vi "_CSM Module Switcher.vi"(7 "Module Name":string="CSM Debug Console") -> ()   [LabVIEW 2017]
uses:
  user.lib/_NEVSTOP/Communicable State Machine(CSM)/_Support/Typedef/_CSM_GlobalLog_MSG.ctl
  user.lib/_NEVSTOP/Communicable State Machine(CSM)/_Support/Typedef/_CSM_Response Source Message.ctl
  user.lib/_NEVSTOP/Communicable State Machine(CSM)/_Support/Typedef/_CSM_GlobalLog_MSG_TYPE.ctl
  user.lib/_NEVSTOP/Communicable State Machine(CSM)/_Support/Common/Format Timestamp.vi
  user.lib/_NEVSTOP/Communicable State Machine(CSM)/AdvanceAPI/CSM - Convert Error to Argument.vi
  user.lib/_NEVSTOP/Communicable State Machine(CSM)/_Support/GlobalEvent/GEvt-Generate with Rule Check.vi
  user.lib/_NEVSTOP/Communicable State Machine(CSM)/AdvanceAPI/CSM - Keywords.vi
  user.lib/_NEVSTOP/Communicable State Machine(CSM)/AdvanceAPI/CSM - Make String Arguments Safe.vi
  user.lib/_NEVSTOP/Communicable State Machine(CSM)/_Support/GlobalEvent/LogFilter/LogFilter - Check.vi
  user.lib/_NEVSTOP/Communicable State Machine(CSM)/_Support/GlobalEvent/Cache-GEvt Refs.vi
  user.lib/_NEVSTOP/Communicable State Machine(CSM)/_Support/GlobalEvent/LogFilter/LogFilter.lvclass
  user.lib/_NEVSTOP/Communicable State Machine(CSM)/Communicable State Machine.lvlib
  user.lib/_NEVSTOP/Communicable State Machine(CSM)/_tool/_jksm/JKISM Message Event.lvlib
  user.lib/_NEVSTOP/Communicable State Machine(CSM)/_csmHelper/API with lvcsm Support/CSM-Helper API with lvcsm Support.lvlib
  user.lib/_NEVSTOP/Communicable State Machine(CSM)/_Shared/CSM Shared.lvlib
panel:
  in  "Toolbar.Exit":bool
  in  "Toolbar.Refresh lvcsm Cache":bool
  in  "Refresh CSMs Button":bool
  in  "CSM":string(combo)
  in  "Toolbar.Open FP":bool
  in  "Toolbar.Open BD":bool
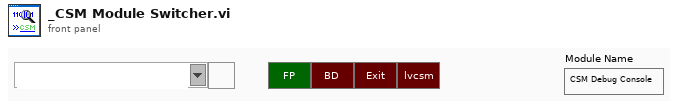
[diagram p1: front panel]
types:
  T1 = typedef "Communicable State Machine.lvlib/_CSM_GlobalLog_MSG.ctl" = cluster{"Name (\"\" to Use UUID)":string, "Current State":string, "Arguments":string, "Source Message":T2, "Source Module":string, "Complete(T)/Start(F)":bool, "LogType":T3, "Time Stamp":timestamp}
  T2 = typedef "Communicable State Machine.lvlib/_CSM_Response Source Message.ctl" = cluster{"‘State":string, "’Arguments":string, "’Error":errorcluster}
  T3 = typedef "Communicable State Machine.lvlib/_CSM_GlobalLog_MSG_TYPE.ctl" = enum16{"User Log", "State Change", "Status", "Interrupt", "Register", "Unregister", "Error Log", "Module Created", "Module Destroyed", "Async Message", "No-Rep Async Message", "Sync Message"}
  T4 = enum32{"Invalid", "Standard", "Closed", "Hidden", "Minimized", "Maximized"}
  T5 = enum32{"invalid app kind", "Development System", "Run Time System", "Student Edition", "Embedded LabVIEW", "Evaluation", "Custom"}
  T6 = cluster{"Shift":bool, "Ctrl":bool, "Alt":bool, "Cmd":bool, "Opt":bool}
  T7 = cluster{"Core":cluster{"Current VI Reference":refnum<vi>, "Close Panel on Exit?":bool}, "lvlps File":path, "Toobar.advance":refnum<vi>[]}
  T8 = cluster{"Current VI Reference":refnum<vi>, "Close Panel on Exit?":bool}
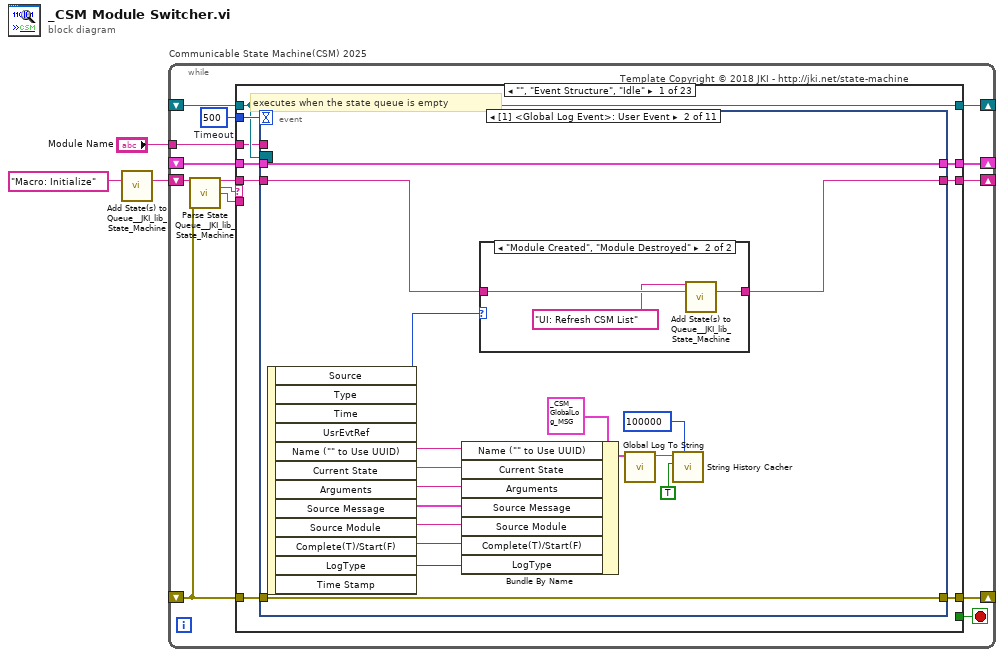
[diagram p0: block diagram]
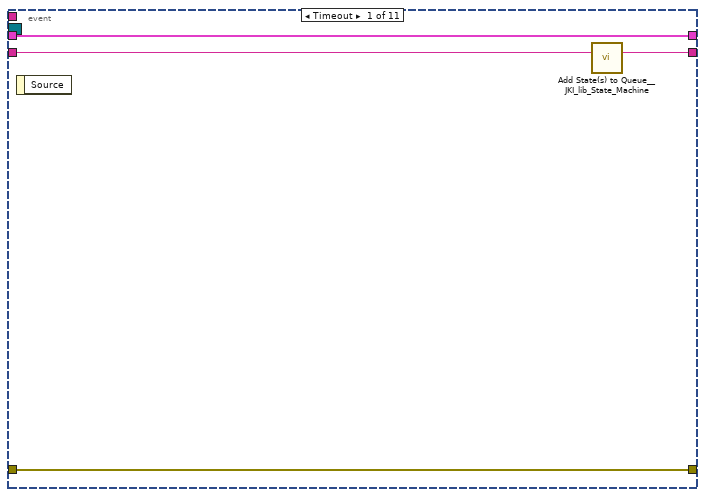
[diagram p2: hidden frame]
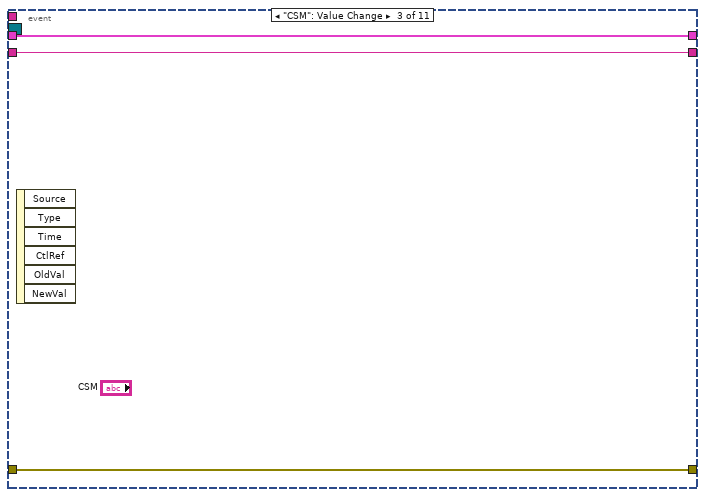
[diagram p4: hidden frame]
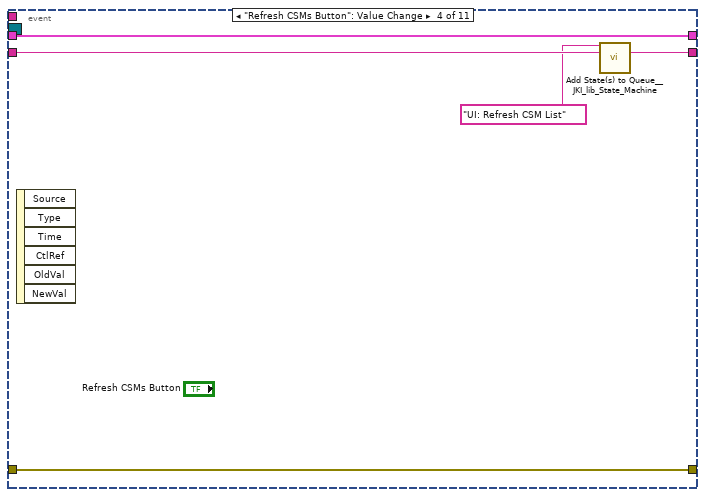
[diagram p5: hidden frame]
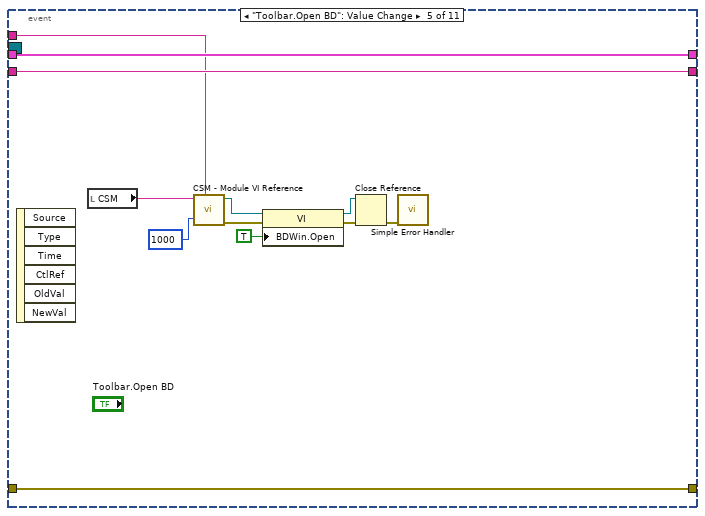
[diagram p6: hidden frame]
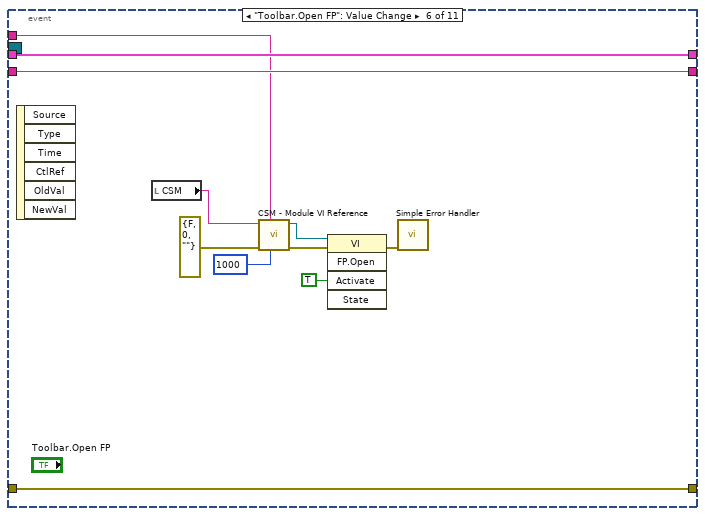
[diagram p7: hidden frame]
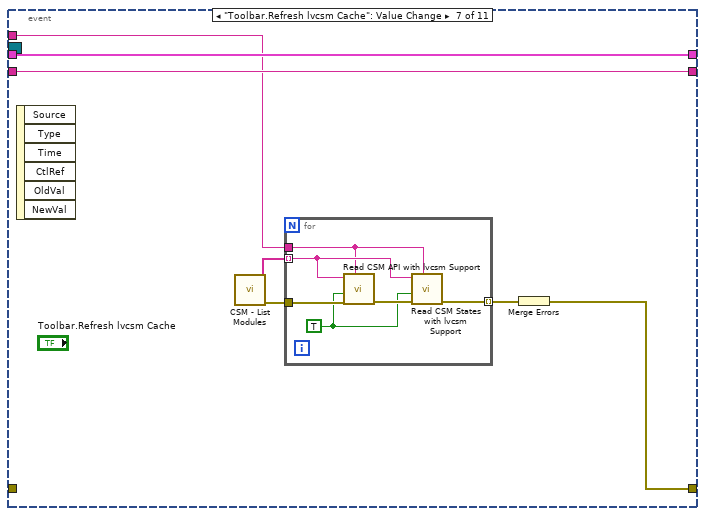
[diagram p8: hidden frame]
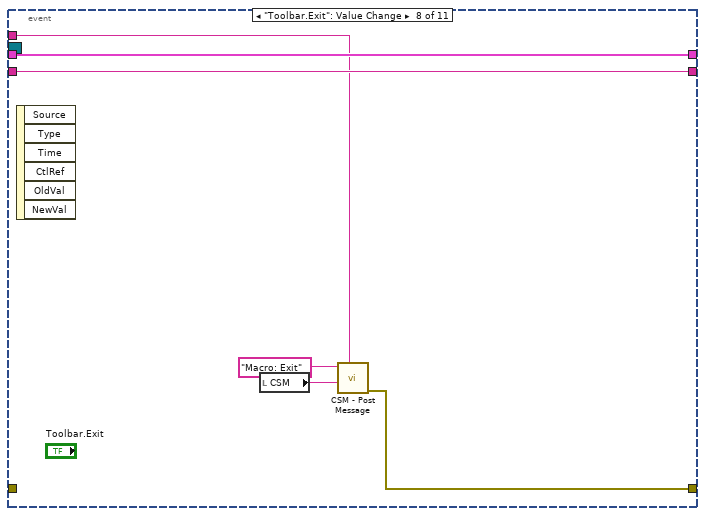
[diagram p9: hidden frame]
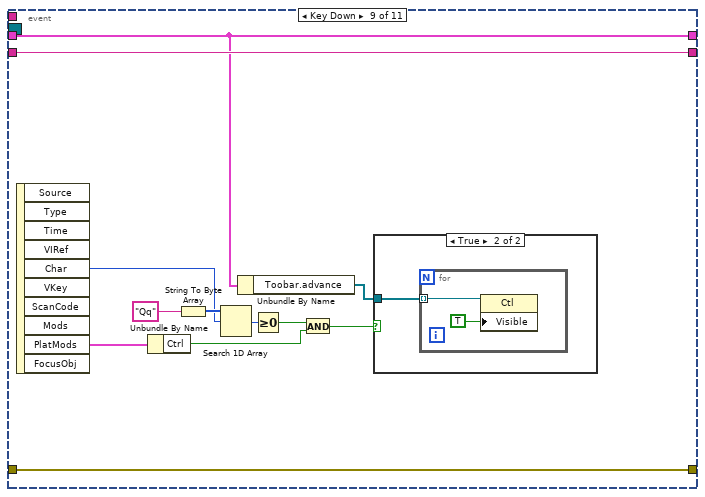
[diagram p10: hidden frame]
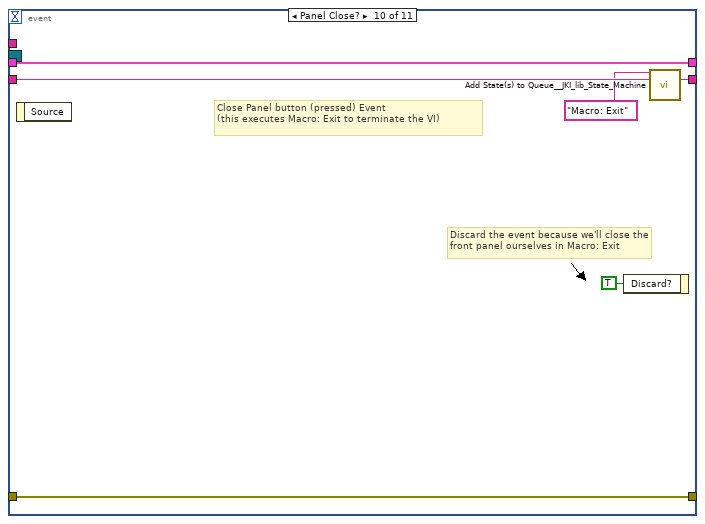
[diagram p12: hidden frame]
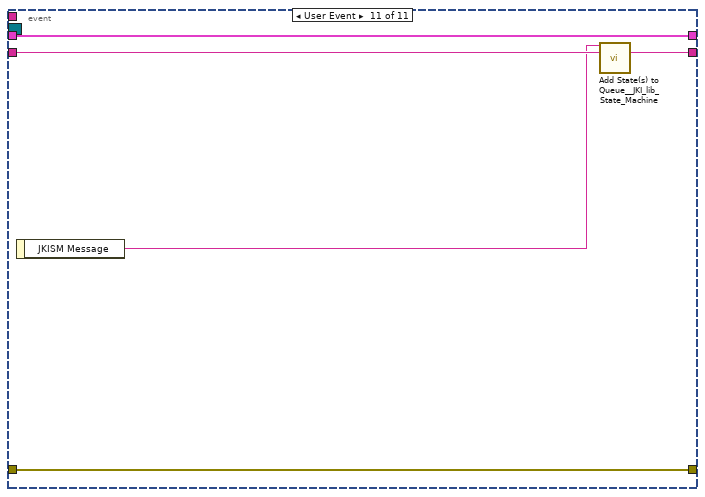
[diagram p13: hidden frame]
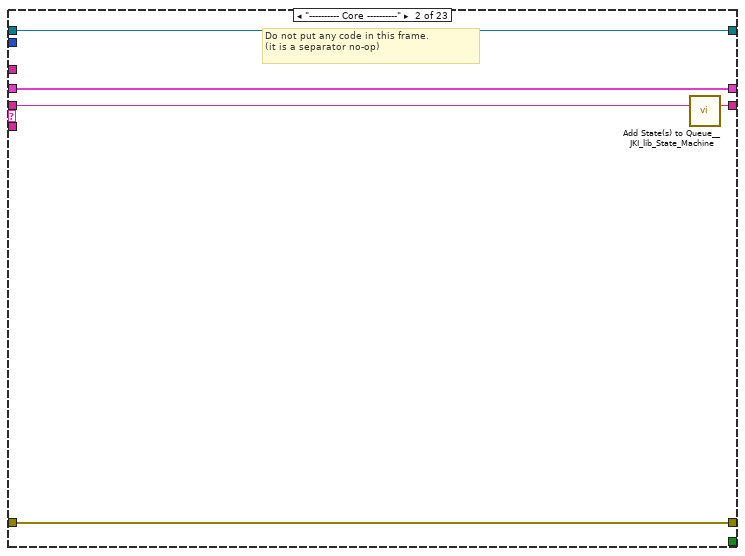
[diagram p14: hidden frame]
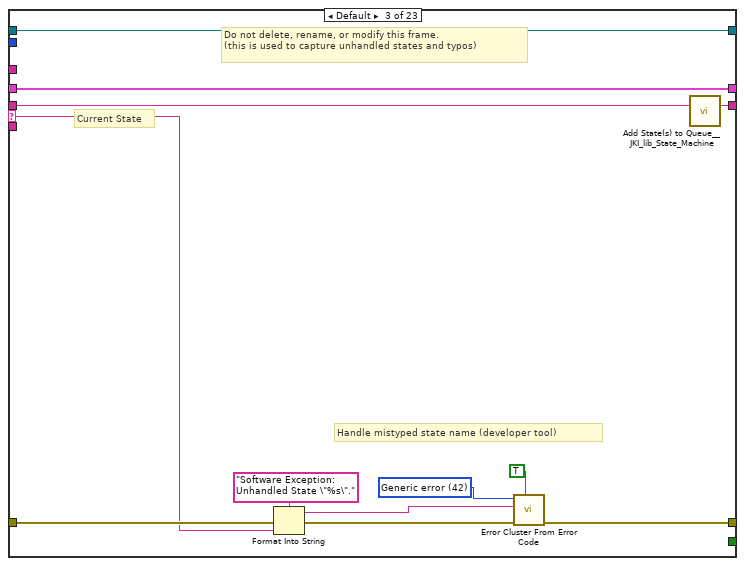
[diagram p15: hidden frame]
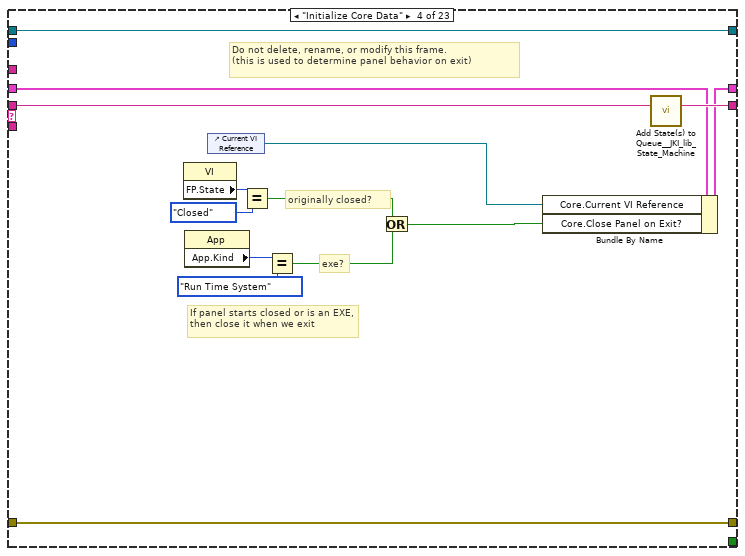
[diagram p16: hidden frame]
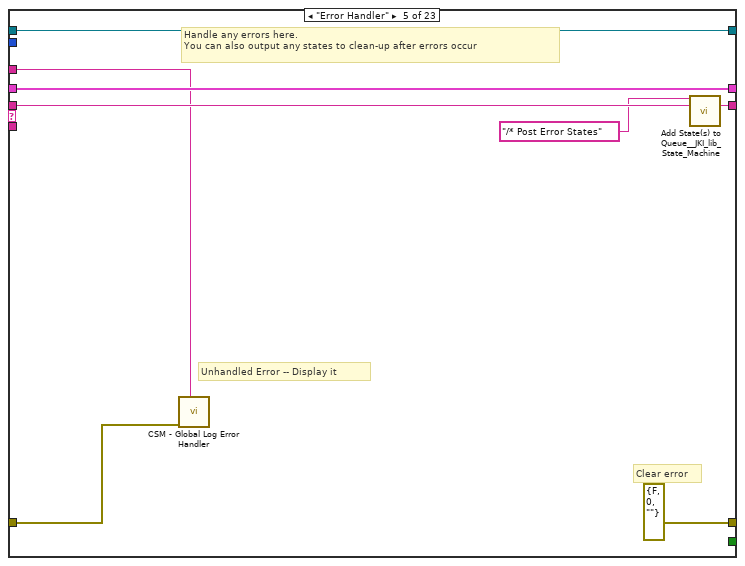
[diagram p17: hidden frame]
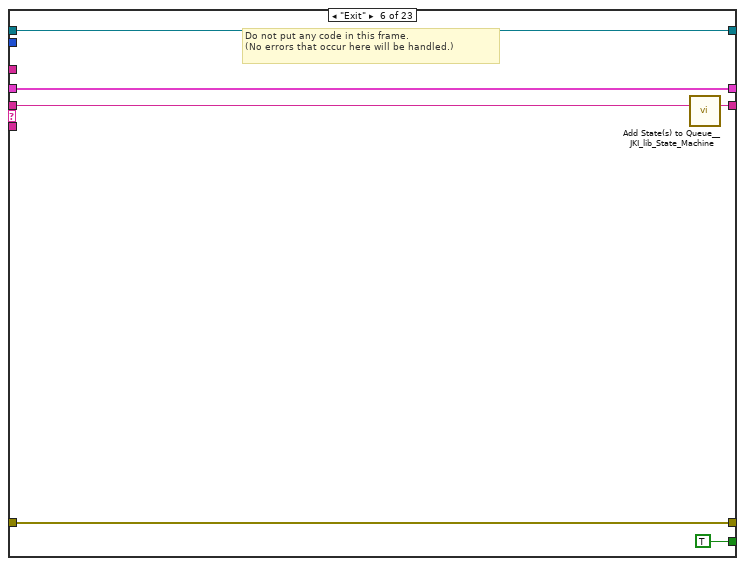
[diagram p18: hidden frame]
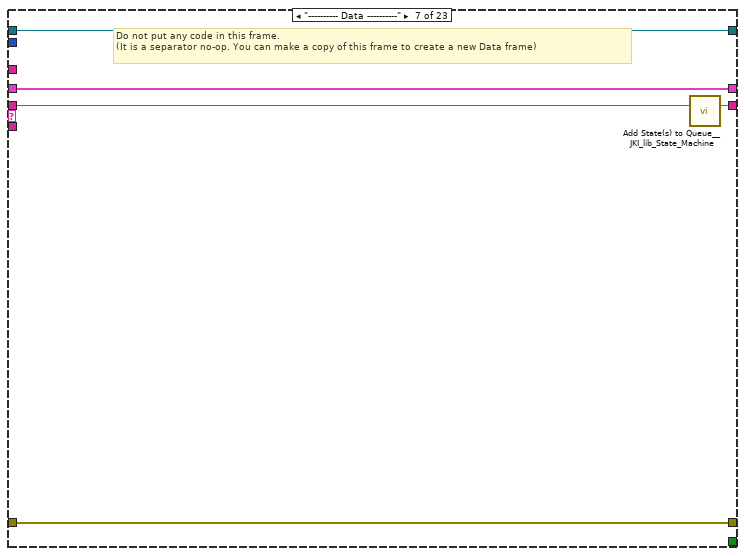
[diagram p19: hidden frame]
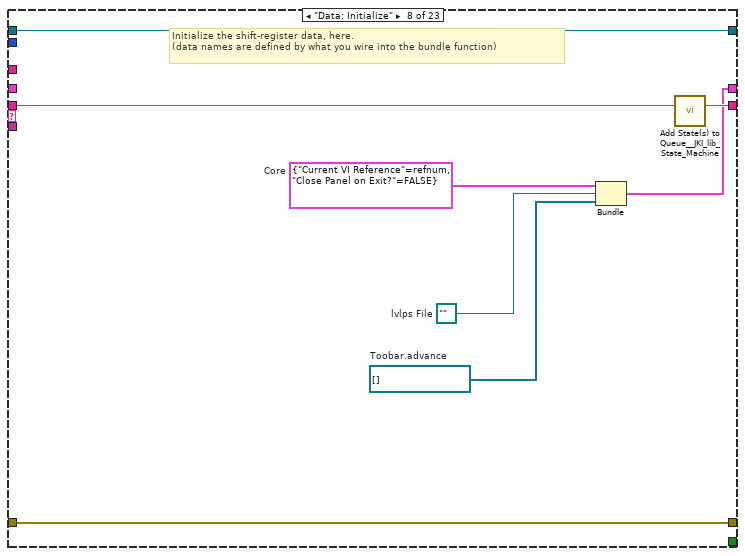
[diagram p20: hidden frame]
diagram:
  n1 = call <vilib>:"Add State(s) to Queue__JKI_lib_State_Machine.vi"("State(s) in (\"\")"="Macro: Initialize") -> ("States Out"=w2:string)  [unwired: 14 in]
  n2 = while "Communicable State Machine(CSM) 2025" {
    shift-right: [w10] -> _
    shift-left: _ -> [w9]
    shift-right: [w13] -> _
    shift-left: _ -> [w7]
    shift-right: [w12] -> _
    shift-left: w2 -> [w14]
    shift-right: [w6] -> _
    shift-left: _ -> [w5]
    tunnel: "Module Name" -> [w4]
    stop <- w11 stop-if-true
    w8 = 500  # Timeout
    # "Template Copyright © 2018 JKI - http://jki.net/state-machine"
    n3 = call <vilib>:"Parse State Queue__JKI_lib_State_Machine.vi"("State Queue"=w14, "Error In (no error)"=w7) -> ("Remaining States"=w16:string, "Current State"=w17:string, "Arguments"=w15:string)  [unwired: 11 in]
    n4 = case shown="\"\", \"Event Structure\", \"Idle\"" w17 {
      selector: w17 -> [_ _ w133 _ _ _ _ _ _ _ _ _ _ _ _ _ _ _ _ _ _ _ _]
      tunnel: w16 -> [w26 w131 w137 w157 w165 w171 w176 w184 w191 w199 w204 w212 w217 w222 w228 w238 w250 w327 w342 w346 w352 w358 w369]
      tunnel: w15 -> [_ _ _ _ _ _ _ _ _ _ _ _ _ _ _ w233 w244 w325 _ _ _ _ _]
      tunnel: w9 -> [w24 w128 w135 w150 w162 w169 w173 _ w190 w194 w201 w210 w213 w219 w224 w236 w246 w322 w341 w344 w349 w355 w366]
      tunnel: [w23 w129 w139 w154 errorcluster {"status"=FALSE, "code"=0, "source"=""} ("error out") w168 w174 w181 w192 w195 w202 w208 w214 w220 w226 w234 w247 w328 w343 w347 w350 w356 w367] -> w13
      tunnel: w7 -> [w22 w129 w138 w154 w161 w168 w174 w181 w192 w196 w202 _ _ w220 w226 w235 w248 w328 w343 w347 w350 w356 w367]
      tunnel: [w25 w130 w136 w156 w164 w170 w175 w183 w191 w198 w203 w211 w216 w221 w227 w237 w249 w327 w342 w346 w351 w357 w368] -> w12
      tunnel: [_ _ _ _ _ TRUE _ _ _ _ _ _ _ _ _ _ _ _ _ _ _ _ _] -> w11
      tunnel: [w21 w128 w135 w155 w162 w169 w173 w182 w186 w194 w201 w210 w213 w219 w224 w236 w246 w322 w341 w344 w349 w355 w366] -> w10
      tunnel: w8 -> [w20 _ _ _ _ _ _ _ _ _ _ _ _ _ _ _ _ _ _ _ _ _ _]
      tunnel: [w19 w127 w132 w144 w159 w166 w172 w179 w189 w193 w200 w209 w215 w218 w225 w232 w243 w326 w340 w345 w348 w353 w359] -> w6
      tunnel: w5 -> [w19 w127 w132 w144 w159 w166 w172 w179 w189 w193 w200 _ w215 w218 w225 w232 w243 w326 w340 w345 w348 w353 w359]
      tunnel: w4 -> [w18 _ _ _ w158 _ _ _ _ _ _ w205 _ _ _ _ _ _ _ _ _ _ _]
      frame "", "Event Structure", "Idle" {
        # "executes when the state queue is empty"
        n5 = event shown="[1] <Global Log Event>: User Event" {
          selector: w19 -> [_ _ _ _ _ _ _ _ _ _ _]
          dyn-events: _ -> [_ _ _ _ _ _ _ _ _ _ _]
          timeout: w20 -> [_ _ _ _ _ _ _ _ _ _ _]
          tunnel: w26 -> [w30 w32 w53 w56 w70 w81 w88 w100 w112 w121 w123]
          tunnel: [w29 w33 w53 w55 w70 w81 w88 w100 w112 w120 w124] -> w25
          tunnel: w24 -> [w27 w45 w51 w57 w69 w80 w87 w99 w101 w118 w125]
          tunnel: [w28 w46 w52 w58 w66 w78 w82 w97 w111 w119 w126] -> w23
          tunnel: w22 -> [w28 w46 w52 w58 w66 w78 _ _ w111 w119 w126]
          tunnel: [w27 w45 w51 w57 w69 w80 w87 w99 w101 w118 w125] -> w21
          tunnel: w18 -> [_ _ _ _ w65 w76 w83 w95 _ _ _]
          event Timeout {
            n6 = event-data() -> ()  [unwired: 1 in, 1 out]
            n7 = call <vilib>:"Add State(s) to Queue__JKI_lib_State_Machine.vi"("State(s) in (\"\")"=w30) -> ("States Out"=w29:string)  [unwired: 14 in]
          }
          event User Event {
            n8 = event-data() -> ("Name (\"\" to Use UUID)"=w39:string, "Current State"=w38:string, "Arguments"=w37:string, "Source Message"=w36:T2, "Source Module"=w35:string, "Complete(T)/Start(F)"=w34:bool, "LogType"=w31:T3)  [unwired: 1 in, 5 out]
            n9 = Bundle By Name(cluster=T1 {"Name (\"\" to Use UUID)"="", "Current State"="", "Arguments"="", "Source Message"={"‘State"="", "’Arguments"="", "’Error"={"status"=FALSE, "code"=0, "source"=""}}, "Source Module"="", "Complete(T)/Start(F)"=FALSE, "LogType"=enum."User Log", "Time Stamp"=timestamp(0 s since 1904-01-01)} ("Cross CSM Data"), "Name (\"\" to Use UUID)"=w39, "Current State"=w38, "Arguments"=w37, "Source Message"=w36, "Source Module"=w35, "Complete(T)/Start(F)"=w34, "LogType"=w31) -> (w44:T1)
            n10 = case shown="\"Module Created\", \"Module Destroyed\"" w31 {
              tunnel: w32 -> [w47 w50]
              tunnel: [w47 w49] -> w33
              frame "User Log", Default {
              }
              frame "Module Created", "Module Destroyed" {
                n11 = call <vilib>:"Add State(s) to Queue__JKI_lib_State_Machine.vi"("State(s) in Front (\"\")"="UI: Refresh CSM List" ("State(s) in Front (\"\")"), "State(s) in (\"\")"=w50) -> ("States Out"=w49:string)  [unwired: 13 in]
              }
            }
            n12 = call "Global Log To String.vi"("Log"=w44) -> ("Log String"=w43:string)  [unwired: 9 in]
            n13 = call "String History Cacher.vi"("Length"=100000 ("length"), "Include Timestamp? (T)"=TRUE ("Include Timestamp(F)"), "String"=w43) -> ()  [unwired: 8 in, 1 out]
          }
          event "CSM": Value Change {
            n14 = event-data() -> ()  [unwired: 1 in, 6 out]
          }
          event "Refresh CSMs Button": Value Change {
            n15 = event-data() -> ()  [unwired: 1 in, 6 out]
            n16 = call <vilib>:"Add State(s) to Queue__JKI_lib_State_Machine.vi"("State(s) in Front (\"\")"="UI: Refresh CSM List" ("State(s) in Front (\"\")"), "State(s) in (\"\")"=w56) -> ("States Out"=w55:string)  [unwired: 13 in]
          }
          event "Toolbar.Open BD": Value Change {
            n17 = event-data() -> ()  [unwired: 1 in, 6 out]
            n18 = local read "CSM"() -> (w67:string)
            n19 = call "CSM - Module VI Reference.vi"("Response Timeout (-2 Using Global Settings)"=1000 ("Response Timeout(5000ms)"), "Current Module (\"\" to Generate an ID)"=w65, "CSM Name"=w67) -> ("error out"=w59:errorcluster, "CSM Module VIRef"=w64:refnum<vi>)  [unwired: 7 in]
            n20 = property class="VI"(reference=w64, error in=w59, "BDWin.Open"=TRUE ("Block Diagram Window:Open")) -> (reference out=w62:refnum<vi>, error out=w61:errorcluster)
            n21 = Close Reference(reference=w62, error in (no error)=w61) -> (error out=w68:errorcluster)
            n22 = call <vilib>:"Simple Error Handler.vi"("error in (no error)"=w68) -> ()  [unwired: 4 in, 5 out]
          }
          event "Toolbar.Open FP": Value Change {
            n23 = event-data() -> ()  [unwired: 1 in, 6 out]
            n24 = local read "CSM"() -> (w79:string)
            n25 = call "CSM - Module VI Reference.vi"("Response Timeout (-2 Using Global Settings)"=1000 ("Response Timeout(5000ms)"), "Current Module (\"\" to Generate an ID)"=w76, "error in (no error)"=errorcluster {"status"=FALSE, "code"=0, "source"=""}, "CSM Name"=w79) -> ("error out"=w72:errorcluster, "CSM Module VIRef"=w73:refnum<vi>)  [unwired: 6 in]
            n26 = invoke on="Invoke Node" class="VI" method="FP.Open"(reference=w73, error in=w72, "Activate"=TRUE ("Activate?")) -> (error out=w77:errorcluster)  [unwired: 2 in, 4 out]
            n27 = call <vilib>:"Simple Error Handler.vi"("error in (no error)"=w77) -> ()  [unwired: 4 in, 5 out]
          }
          event "Toolbar.Refresh lvcsm Cache": Value Change {
            n28 = event-data() -> ()  [unwired: 1 in, 6 out]
            n29 = call "CSM - List Modules.vi"() -> ("error out"=w86:errorcluster, "Module Names"=w85:string[])  [unwired: 10 in]
            n30 = for {
              tunnel: w86 -> [w94]
              tunnel: w85 -> [w92] mode=indexing
              tunnel: w83 -> [w91]
              tunnel: [w90] -> w84 mode=indexing
              w89 = TRUE ("Force?(F)")
              n31 = call "Read CSM API with lvcsm Support.vi"("Current Module (\"\" to Generate an ID)"=w91, "error in (no error)"=w94, "Force? (F)"=w89, "CSM Name"=w92) -> ("error out"=w93:errorcluster)  [unwired: 6 in, 1 out]
              n32 = call "Read CSM States with lvcsm Support.vi"("Current Module (\"\" to Generate an ID)"=w91, "error in (no error)"=w93, "Force? (F)"=w89, "CSM Name"=w92) -> ("error out"=w90:errorcluster)  [unwired: 6 in, 1 out]
            }
            n33 = Merge Errors(w84) -> (w82:errorcluster)
          }
          event "Toolbar.Exit": Value Change {
            n34 = event-data() -> ()  [unwired: 1 in, 6 out]
            n35 = local read "CSM"() -> (w98:string)
            n36 = call "CSM - Post Message.vi"("Current Module (\"\" to Generate an ID)"=w95, "Target Module"=w98, "State"="Macro: Exit") -> ("error out"=w97:errorcluster)  [unwired: 8 in]
          }
          event Key Down {
            n37 = event-data() -> ("Char"=w102:i16, "PlatMods"=w103:T6)  [unwired: 1 in, 8 out]
            n38 = Unbundle By Name(w103) -> ("Ctrl"=w106:bool)
            n39 = String To Byte Array(string="Qq") -> (unsigned byte array=w108:u8[])
            n40 = Search 1D Array(1D array=w108, element=w102) -> (index of element=w109:i32)  [unwired: 1 in]
            n41 = Unbundle By Name(w101) -> ("Toobar.advance"=w104:refnum<vi>[])
            n42 = Greater Or Equal To 0?(x=w109) -> (x >= 0?=w110:bool)
            n43 = And(x=w110, y=w106) -> (x .and. y?=w105:bool)
            n44 = case shown="True" w105 {
              tunnel: w104 -> [_ w113]
              frame False {
              }
              frame True {
                n45 = for {
                  tunnel: w113 -> [w115] mode=indexing
                  n46 = property class="Ctl"(reference=w115, "Visible"=TRUE) -> ()  [unwired: 1 in, 2 out]
                }
              }
            }
          }
          event Panel Close? {
            # "Discard the event because we'll close the front panel ourselves in Macro: Exit"
            # "Close Panel button (pressed) Event\n(this executes Macro: Exit to terminate the VI)"
            n47 = event-data() -> ()  [unwired: 1 in, 1 out]
            n48 = event-data("Discard?"=TRUE) -> ()  [unwired: 1 in, 1 out]
            n49 = call <vilib>:"Add State(s) to Queue__JKI_lib_State_Machine.vi"("State(s) in Front (\"\")"="Macro: Exit", "State(s) in (\"\")"=w121) -> ("States Out"=w120:string)  [unwired: 13 in]
          }
          event User Event {
            n50 = event-data() -> ("JKISM Message"=w122:string)  [unwired: 1 in]
            n51 = call <vilib>:"Add State(s) to Queue__JKI_lib_State_Machine.vi"("State(s) in Front (\"\")"=w122, "State(s) in (\"\")"=w123) -> ("States Out"=w124:string)  [unwired: 13 in]
          }
        }
      }
      frame "---------- Core ----------" {
        # "Do not put any code in this frame.\n(it is a separator no-op)"
        n52 = call <vilib>:"Add State(s) to Queue__JKI_lib_State_Machine.vi"("State(s) in (\"\")"=w131) -> ("States Out"=w130:string)  [unwired: 14 in]
      }
      frame Default {
        w142 = 42 items=["No error", "Argument error", "Memory is full", "Out of zone", "End of file", "File already open", "Generic file I/O error", "File not found", "File permission error", "Disk is full", "Duplicate path", "Too many files open", "System feature not enabled", "Resource file not found", "Cannot add resource", "Resource not found", "Image not found", "Image memory error", "Pen does not exist", "Config type invalid", "Config token not found", "Config parse error", "Config memory error", "Bad external code format", "Bad external code offset", "External code not present", "Null window", "Destroy window error", "Null menu", "Print aborted", "Bad print record", "Print driver error", "Windows error during printing", "Memory error during printing", "Print dialog error", "Generic print error", "Invalid device refnum", "Device not found", "Device parameter error", "Device unit error", "Cannot open device", "Device call aborted", "Generic error", "Cancelled by user", "Object ID too low", "Object ID too high", "Object not in heap", "Unknown heap", "Unknown object (invalid DefProc)", "Unknown object (DefProc not in table)", "Message out of range", "Invalid (null) method", "Unknown message", "Manager call not supported", "Bad address", "Network operation in progress", "Network operation timed out", "Connection is busy", "Network attribute not supported", "Network error", "Address in use", "System out of memory", "Connection aborted", "Connection refused", "Not connected", "Already connected", "Connection closed", "Initialization error (interapplication manager)", "Bad occurrence", "Wait on unbound occurrence handler", "Occurrence queue overflow", "Datalog type conflict", "Unused", "Unrecognized type (interapplication manager)", "Memory corrupt", "Failed to make temporary DLL", "Old CIN version", "Drag socket not found", "Failed to load drop-object", "Failed to register OLE object", "Failed to release OLE object", "Format specifier type mismatch", "Unknown format specifier", "Too few format specifiers", "Too many format specifiers", "Scan failed", "Newer CIN version", "Error converting to variant", "Runtime menu error", "Password tampered", "Variant attribute not found", "Incompatible variant data type", "Event data is not available", "Event Store is not present", "Occurrence is not found", "Event Queue is not created", "Event info is not available", "Refnum passed is NULL", "Error retrieving Class GUID", "Error retrieving CoClass GUID", "Error retrieving TypeLib GUID.", "Bad built application magic bytes.", "Specific driver is different from the specific driver associated with the Logical Name.", "There is no session opened to the class driver.", "Max Error", "MAX - Error with config objects", "MAX - Error loading configuration", "MAX - Group not supported"]
        # "Current State"
        # "Do not delete, rename, or modify this frame.\n(this is used to capture unhandled states and typos)"
        # "Handle mistyped state name (developer tool)"
        n53 = Format Into String(format string="Software Exception: Unhandled State \"%s\"." ("message"), error in=w138, w133) -> (resulting string=w141:string, error out=w140:errorcluster)  [unwired: 1 in]
        n54 = call <vilib>:"Error Cluster From Error Code.vi"("show call chain? (False)"=TRUE, "error in (no error)"=w140, "error message (\"\")"=w141, "error code (0)"=w142) -> ("error out"=w139:errorcluster)  [unwired: 5 in]
        n55 = call <vilib>:"Add State(s) to Queue__JKI_lib_State_Machine.vi"("State(s) in (\"\")"=w137) -> ("States Out"=w136:string)  [unwired: 14 in]
      }
      frame "Initialize Core Data" {
        # "Do not delete, rename, or modify this frame.\n(this is used to determine panel behavior on exit)"
        # "originally closed?"
        # "exe?"
        # "If panel starts closed or is an EXE, then close it when we exit"
        n56 = property class="VI"() -> ("FP.State"=w147:T4)  [unwired: 2 in, 2 out]
        n57 = property class="App"() -> ("App.Kind"=w153:T5)  [unwired: 2 in, 2 out]
        n58 = control-ref of="Current VI Reference"() -> (w148:refnum<vi>)
        n59 = Equal?(x=w147, y=T4."Closed" ("Front Panel Window:State")) -> (x = y?=w145:bool)
        n60 = Equal?(x=w153, y=T5."Run Time System" ("Application:Kind")) -> (x = y?=w151:bool)
        n61 = Or(x=w145, y=w151) -> (x .or. y?=w149:bool)
        n62 = Bundle By Name(cluster=w150, "Core.Current VI Reference"=w148, "Core.Close Panel on Exit?"=w149) -> (w155:T7)
        n63 = call <vilib>:"Add State(s) to Queue__JKI_lib_State_Machine.vi"("State(s) in (\"\")"=w157) -> ("States Out"=w156:string)  [unwired: 14 in]
      }
      frame "Error Handler" {
        # "Unhandled Error -- Display it"
        # "Handle any errors here.\nYou can also output any states to clean-up after errors occur"
        # "Clear error"
        n64 = call "CSM - Global Log Error Handler.vi"("Place (\"\" to Use VI's Name)"=w158, "Error In"=w161) -> ()  [unwired: 9 in, 1 out]
        n65 = call <vilib>:"Add State(s) to Queue__JKI_lib_State_Machine.vi"("State(s) in Front (\"\")"="/* Post Error States", "State(s) in (\"\")"=w165) -> ("States Out"=w164:string)  [unwired: 13 in]
      }
      frame "Exit" {
        # "Do not put any code in this frame.\n(No errors that occur here will be handled.)"
        n66 = call <vilib>:"Add State(s) to Queue__JKI_lib_State_Machine.vi"("State(s) in (\"\")"=w171) -> ("States Out"=w170:string)  [unwired: 14 in]
      }
      frame "---------- Data ----------" {
        # "Do not put any code in this frame.\n(It is a separator no-op. You can make a copy of this frame to create a new Data frame)"
        n67 = call <vilib>:"Add State(s) to Queue__JKI_lib_State_Machine.vi"("State(s) in (\"\")"=w176) -> ("States Out"=w175:string)  [unwired: 14 in]
      }
      frame "Data: Initialize" {
        w177 = refnum<vi>[] []  # Toobar.advance
        w178 = path ""  # lvlps File
        w180 = T8 {"Current VI Reference"=refnum, "Close Panel on Exit?"=FALSE}  # Core
        # "Initialize the shift-register data, here.\n(data names are defined by what you wire into the bundle function)"
        n68 = Bundle("Core"=w180, "lvlps File"=w178, "Toobar.advance"=w177) -> (w182:T7)  [unwired: 1 in]
        n69 = call <vilib>:"Add State(s) to Queue__JKI_lib_State_Machine.vi"("State(s) in (\"\")"=w184) -> ("States Out"=w183:string)  [unwired: 14 in]
      }
      frame "Data: Initialize References" {
        n70 = control-ref of="Toolbar.Open FP"() -> (w188:refnum<vi>)
        n71 = control-ref of="Toolbar.Open BD"() -> (w187:refnum<vi>)
        n72 = Build Array(w188, w187) -> (w185:refnum<vi>[])
        n73 = Bundle By Name(cluster=w190, "Toobar.advance"=w185) -> (w186:T7)
      }
      frame "Data: Cleanup" {
        # "Cleanup any data and references, here.\n(this is called automatically, by the Macro: Exit)"
        n74 = Unbundle By Name(w194) -> ("Core.Current VI Reference"=w197:refnum<vi>)
        n75 = Close Reference(reference=w197, error in (no error)=w196) -> (error out=w195:errorcluster)
        n76 = call <vilib>:"Add State(s) to Queue__JKI_lib_State_Machine.vi"("State(s) in (\"\")"=w199) -> ("States Out"=w198:string)  [unwired: 14 in]
      }
      frame "---------- Events ----------" {
        # "Do not put any code in this frame.\n(It is a separator no-op. You can make a copy of this frame to create a new UI frame)"
        n77 = call <vilib>:"Add State(s) to Queue__JKI_lib_State_Machine.vi"("State(s) in (\"\")"=w204) -> ("States Out"=w203:string)  [unwired: 14 in]
      }
      frame "Events: Register" {
        # "Do not put any code in this frame.\n(It is a separator no-op. You can make a copy of this frame to create a new UI frame)"
        n78 = call "CSM - Global Log Event.vi"() -> ("Global Log Event"=w207:refnum<user-event>)  [unwired: 10 in, 1 out]
        n79 = call "Obtain JKISM Message Event.vi"("Module"=w205) -> ("JKISM Message Event"=w206:refnum<user-event>)  [unwired: 9 in, 1 out]
        n80 = register-events(w207, w206) -> (reference out=w209:refnum<event-registration>, error out=w208:errorcluster)  [unwired: 2 in]
        n81 = call <vilib>:"Add State(s) to Queue__JKI_lib_State_Machine.vi"("State(s) in (\"\")"=w212) -> ("States Out"=w211:string)  [unwired: 14 in]
      }
      frame "Events: Unregister" {
        # "Do not put any code in this frame.\n(It is a separator no-op. You can make a copy of this frame to create a new UI frame)"
        n82 = Unregister For Events(event registration refnum=w215) -> (error out=w214:errorcluster)  [unwired: 1 in]
        n83 = call <vilib>:"Add State(s) to Queue__JKI_lib_State_Machine.vi"("State(s) in (\"\")"=w217) -> ("States Out"=w216:string)  [unwired: 14 in]
      }
      frame "---------- UI ----------" {
        # "Do not put any code in this frame.\n(It is a separator no-op. You can make a copy of this frame to create a new UI frame)"
        n84 = call <vilib>:"Add State(s) to Queue__JKI_lib_State_Machine.vi"("State(s) in (\"\")"=w222) -> ("States Out"=w221:string)  [unwired: 14 in]
      }
      frame "UI: Initialize" {
        # "Initialize the User Interface, here.\n(this is called automatically, by the Macro: Init)"
        n85 = Unbundle By Name(w224) -> ("Toobar.advance"=w223:refnum<vi>[])
        n86 = disable-structure shown="Disabled" {
          disable-tunnel: w223 -> [w229 _]
          frame Disabled {
            n87 = for {
              tunnel: w229 -> [w231] mode=indexing
              n88 = property class="Ctl"(reference=w231, "Visible"=FALSE) -> ()  [unwired: 1 in, 2 out]
            }
          }
          frame Enabled {
          }
        }
        n89 = call <vilib>:"Add State(s) to Queue__JKI_lib_State_Machine.vi"("State(s) in (\"\")"=w228) -> ("States Out"=w227:string)  [unwired: 14 in]
      }
      frame "UI: Cursor Set" {
        # "Argument"
        # "Set and Unset Cursor Busy.\n(Usage: \"UI: Cursor Set >> Busy|Idle\")"
        n90 = case shown="\"Idle\", Default" w233 {
          tunnel: w235 -> [w240 w242]
          tunnel: [w239 w241] -> w234
          frame "Idle", Default {
            n91 = call <vilib>:"Unset Busy.vi"("error in (no error)"=w240) -> ("error out"=w239:errorcluster)  [unwired: 10 in]
          }
          frame "Busy" {
            n92 = call <vilib>:"Set Busy.vi"("error in (no error)"=w242) -> ("error out"=w241:errorcluster)  [unwired: 9 in, 1 out]
          }
        }
        n93 = call <vilib>:"Add State(s) to Queue__JKI_lib_State_Machine.vi"("State(s) in (\"\")"=w238) -> ("States Out"=w237:string)  [unwired: 14 in]
      }
      frame "UI: Front Panel State" {
        # "Argument"
        # "Set Front Panel Open or Closed\n(Usage: \"UI: Front Panel State >> Open|Close\")"
        n94 = Unbundle By Name(w246) -> ("Core.Current VI Reference"=w245:refnum<vi>)
        n95 = case shown="\"Minimize\", \"Minimized\"" w244 {
          tunnel: w248 -> [w256 w271 w282 w295 w308]
          tunnel: [w258 w272 w284 w297 w310] -> w247
          tunnel: w245 -> [w257 w269 w283 w296 w309]
          frame "Open", "Standard", Default {
            w251 = T4."Standard" ("State")
            n96 = property class="VI"(reference=w257, error in=w256) -> (reference out=w254:refnum<vi>, error out=w255:errorcluster, "FP.State"=w253:T4)
            n97 = Not Equal?(x=w253, y=w251) -> (x != y?=w252:bool)
            n98 = case shown="True" w252 {
              tunnel: [w262 w264] -> w258
              tunnel: w255 -> [w261 w264]
              tunnel: w254 -> [w260 _]
              tunnel: w251 -> [w259 _]
              frame True {
                n99 = invoke class="VI" method="FP.Open"(reference=w260, error in=w261, "Activate"=TRUE, "State"=w259) -> (error out=w262:errorcluster)  [unwired: 1 in, 4 out]
              }
              frame False {
              }
            }
          }
          frame "Close", "Closed" {
            n100 = property class="VI"(reference=w269, error in=w271) -> (reference out=w268:refnum<vi>, error out=w270:errorcluster, "FP.State"=w266:T4)
            n101 = Not Equal?(x=w266, y=T4."Closed" ("Front Panel Window:State")) -> (x != y?=w265:bool)
            n102 = case shown="True" w265 {
              tunnel: [w273 w276] -> w272
              tunnel: w270 -> [w273 w275]
              tunnel: w268 -> [_ w274]
              frame False {
              }
              frame True {
                n103 = invoke class="VI" method="FP.Close"(reference=w274, error in=w275) -> (error out=w276:errorcluster)  [unwired: 1 in, 2 out]
              }
            }
          }
          frame "Hidden", "Hide" {
            w277 = T4."Hidden" ("State")
            n104 = property class="VI"(reference=w283, error in=w282) -> (reference out=w280:refnum<vi>, error out=w281:errorcluster, "FP.State"=w279:T4)
            n105 = Not Equal?(x=w279, y=w277) -> (x != y?=w278:bool)
            n106 = case shown="True" w278 {
              tunnel: [w288 w289] -> w284
              tunnel: w281 -> [w287 w289]
              tunnel: w280 -> [w286 _]
              tunnel: w277 -> [w285 _]
              frame True {
                n107 = invoke class="VI" method="FP.Open"(reference=w286, error in=w287, "State"=w285) -> (error out=w288:errorcluster)  [unwired: 2 in, 4 out]
              }
              frame False {
              }
            }
          }
          frame "Minimize", "Minimized" {
            w290 = T4."Minimized" ("State")
            n108 = property class="VI"(reference=w296, error in=w295) -> (reference out=w293:refnum<vi>, error out=w294:errorcluster, "FP.State"=w292:T4)
            n109 = Not Equal?(x=w292, y=w290) -> (x != y?=w291:bool)
            n110 = case shown="True" w291 {
              tunnel: [w301 w302] -> w297
              tunnel: w294 -> [w300 w302]
              tunnel: w293 -> [w299 _]
              tunnel: w290 -> [w298 _]
              frame True {
                n111 = invoke class="VI" method="FP.Open"(reference=w299, error in=w300, "State"=w298) -> (error out=w301:errorcluster)  [unwired: 2 in, 4 out]
              }
              frame False {
              }
            }
          }
          frame "Maximize", "Maximized" {
            w303 = T4."Maximized" ("State")
            n112 = property class="VI"(reference=w309, error in=w308) -> (reference out=w306:refnum<vi>, error out=w307:errorcluster, "FP.State"=w305:T4)
            n113 = Not Equal?(x=w305, y=w303) -> (x != y?=w304:bool)
            n114 = case shown="True" w304 {
              tunnel: [w314 w315] -> w310
              tunnel: w307 -> [w313 w315]
              tunnel: w306 -> [w312 _]
              tunnel: w303 -> [w311 _]
              frame True {
                n115 = invoke class="VI" method="FP.Open"(reference=w312, error in=w313, "State"=w311) -> (error out=w314:errorcluster)  [unwired: 2 in, 4 out]
              }
              frame False {
              }
            }
          }
        }
        n116 = call <vilib>:"Add State(s) to Queue__JKI_lib_State_Machine.vi"("State(s) in (\"\")"=w250) -> ("States Out"=w249:string)  [unwired: 14 in]
      }
      frame "UI: Autoset Arguments" {
        n117 = call "CSM - Revert Arguments-Safe String.vi"("Safe Argument String"=w325) -> ("Origin Argument String"=w323:string)  [unwired: 8 in]
        n118 = control-ref of="CSM"() -> (w321:refnum<vi>)
        n119 = call "Remove Comments from Single-line.vi"("single-line text"=w323) -> ("single-line text without comments"=w324:string)  [unwired: 2 in]
        n120 = call "Split Single-line Message.vi"("single-line text"=w324) -> ("source/target"=w318:string)  [unwired: 6 in, 3 out]
        n121 = property on="Property Node" class="CmbBox"(reference=w321) -> (reference out=w319:refnum<vi>, "Strings[]"=w320:string[])  [unwired: 1 in, 1 out]
        n122 = Search 1D Array(1D array=w320, element=w318) -> (index of element=w317:i32)  [unwired: 1 in]
        n123 = Greater Or Equal To 0?(x=w317) -> (x >= 0?=w316:bool)
        n124 = case shown="False" w316 {
          tunnel: w319 -> [_ w330]
          tunnel: w318 -> [_ w329]
          frame False {
          }
          frame True {
            n125 = property on="Property Node" class="CmbBox"(reference=w330, "Value"=w329) -> ()  [unwired: 1 in, 2 out]
          }
        }
      }
      frame "UI: Refresh CSM List" {
        n126 = control-ref of="CSM"() -> (w339:refnum<vi>)
        n127 = property on="Property Node" class="CmbBox"(reference=w339) -> (reference out=w331:refnum<vi>, "Value"=w335:string)  [unwired: 1 in, 1 out]
        n128 = call "CSM - List Modules.vi"() -> ("error out"=w338:errorcluster, "Module Names"=w333:string[])  [unwired: 10 in]
        n129 = Search 1D Array(1D array=w333, element=w335) -> (index of element=w337:i32)  [unwired: 1 in]
        n130 = Greater Or Equal To 0?(x=w337) -> (x >= 0?=w336:bool)
        n131 = Index Array(array=w333) -> (element=w334:string)  [unwired: 1 in]
        n132 = Select(t=w335, s=w336, f=w334) -> (s? t:f=w332:string)
        n133 = property on="Property Node" class="CmbBox"(reference=w331, "Strings[]"=w333, "Value"=w332) -> ()  [unwired: 1 in, 2 out]
        n134 = call <vilib>:"Simple Error Handler.vi"("error in (no error)"=w338) -> ()  [unwired: 4 in, 5 out]
      }
      frame "UI: Refresh UI" {
      }
      frame "---------- Macro ----------" {
        # "Do not put any code in this frame.\n(It is a separator no-op. You can make a copy of this frame to create a new Macro frame)"
        n135 = call <vilib>:"Add State(s) to Queue__JKI_lib_State_Machine.vi"("State(s) in (\"\")"=w352) -> ("States Out"=w351:string)  [unwired: 14 in]
      }
      frame "Macro: Initialize" {
        # "Initialization Macro\n(This is called once, when the VI starts)"
        n136 = call <vilib>:"Add State(s) to Queue__JKI_lib_State_Machine.vi"("State(s) in Front (\"\")"="Data: Initialize\nData: Initialize References\nInitialize Core Data\nEvents: Register\nUI: Initialize\nUI: Front Panel State >> Open\nUI: Refresh CSM List\nUI: Refresh UI", "State(s) in (\"\")"=w358) -> ("States Out"=w357:string)  [unwired: 13 in]
      }
      frame "Macro: Exit" {
        # "Exit Macro\n(This is called once, when the VI exits)"
        n137 = Unbundle By Name(w366) -> ("Core.Close Panel on Exit?"=w365:bool)
        n138 = Select(t="UI: Front Panel State >> Close", s=w365, f="") -> (s? t:f=w362:string)
        n139 = call <vilib>:"Add State(s) to Queue__JKI_lib_State_Machine.vi"("State(s) in (\"\")"=w362, "State(s) at Back (\"\")"="Data: Cleanup\nEvents: Unregister\nExit") -> ("States Out"=w360:string)  [unwired: 13 in]
        n140 = call <vilib>:"Add State(s) to Queue__JKI_lib_State_Machine.vi"("State(s) in Front (\"\")"=w360, "State(s) in (\"\")"=w369) -> ("States Out"=w368:string)  [unwired: 13 in]
      }
    }
  }
